vi "log.vi"(8 "error in (no error)":errorcluster, 10 "logLineIn":string, 11 "Protocol_Generic in":refnum<class "Protocol_Generic.lvclass">) -> (0 "error out":errorcluster, 3 "Protocol_Generic out":refnum<class "Protocol_Generic.lvclass">)   [LabVIEW 2015, in "Protocol_Generic.lvclass"]
uses:
  Protocol_Generic.lvclass
  Protocol_Generic.lvclass/Protocol_Generic.ctl
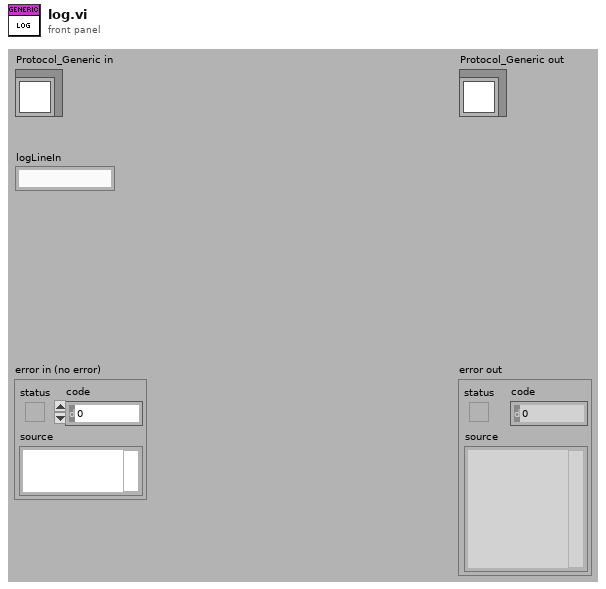
[diagram p1: front panel]
types:
  T1 = enum16{"open", "replace", "create", "open or create", "replace or create", "replace or create with confirmation"}
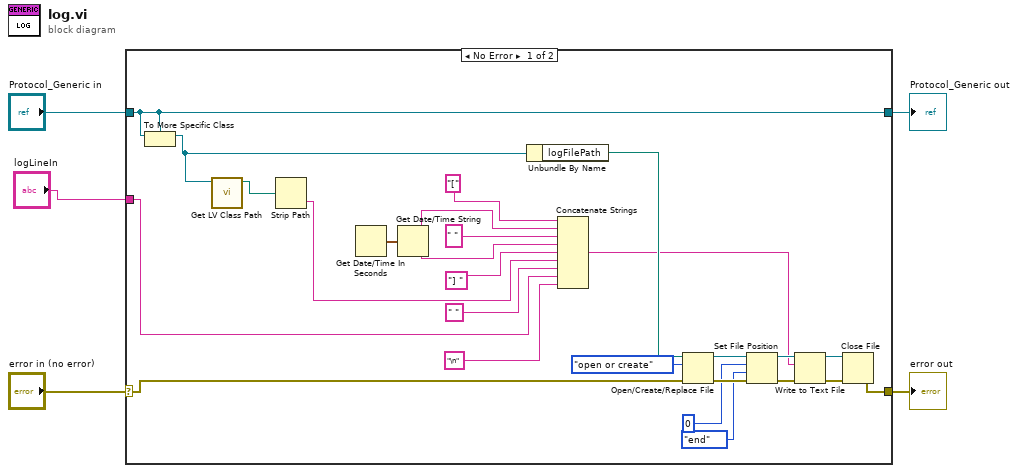
[diagram p0: block diagram]
diagram:
  n1 = case shown="No Error" "error in (no error)" {
    selector: "error in (no error)" -> [w9 w33]
    tunnel: [w24 w33] -> w4
    tunnel: [w8 w32] -> w2
    tunnel: "Protocol_Generic in" -> [w8 w32]
    tunnel: "logLineIn" -> [w12 _]
    frame No Error {
      n2 = To More Specific Class(target class=w8, reference=w8) -> (specific class reference=w7:refnum<class "Protocol_Generic.lvclass">)  [unwired: 1 in, 1 out]
      n3 = call <vilib>:"Get LV Class Path.vi"("object"=w7) -> ("class path"=w14:path)  [unwired: 9 in, 1 out]
      n4 = Strip Path(path=w14) -> (name=w13:string)  [unwired: 1 out]
      n5 = Get Date/Time In Seconds() -> (seconds since 1Jan1904=w21:timestamp)
      n6 = Get Date/Time String(seconds (now)=w21) -> (date string=w17:string, time string=w19:string)  [unwired: 2 in]
      n7 = Unbundle By Name(w7) -> ("logFilePath"=w31:path)
      n8 = Concatenate Strings("[" ("string"), w17, " " ("string"), w19, "] " ("string"), w13, " " ("string"), w12, "\n" ("string")) -> (w20:string)
      n9 = Open/Create/Replace File(file path (use dialog)=w31, error in=w9, operation (0:open)=T1."open or create") -> (refnum out=w28:refnum<file>, error out=w30:errorcluster)  [unwired: 3 in, 1 out]
      n10 = Set File Position(offset (in bytes) (0)=i64 0, refnum=w28, from (0:start)=enum16{"start", "end", "current"}."end", error in=w30) -> (refnum out=w27:refnum<file>, error out=w29:errorcluster)
      n11 = Write to Text File(file (use dialog)=w27, text=w20, error in=w29) -> (refnum out=w23:refnum<file>, error out=w25:errorcluster)  [unwired: 1 in, 1 out]
      n12 = Close File(refnum=w23, error in=w25) -> (error out=w24:errorcluster)  [unwired: 1 out]
    }
    frame Error {
    }
  }
  "error out" <- w4
  "Protocol_Generic out" <- w2
